vi "GUI.vi"() -> ()   [LabVIEW 2020]
uses:
  Sensor910/Sensor910.lvclass
  <vilib>/Utility/miscctls.llb/LVRectTypeDef.ctl
  Sensor910/Settings.ctl
  Sensor910/Mode.ctl
  Sensor910/Command.ctl
panel:
  in  "View Square":bool
  out "График температуры":sgl(graph)
  out "Connection":bool caption="Подключение"
  out "Tab Control":enum32{"Параметры", "Работа"}(tab)
  in  "h reg":u16=48 caption="Регистр h"
  in  "Modbus h":u8=240 caption="Адрес Modbus (Эталон H)"
  in  "dopusk":sgl=0.2 caption="Допуск погрешности, °С"
  in  "Temp Register 2":u8=2 caption="Регистр t (Эталон Т)"
  in  "Period":i64=100 caption="Частота опроса, мс"
  in  "Modbus t":u8=200 caption="Адрес Modbus (Эталон Т)"
  in  "Baud Rate":u32(ring)=9600 caption="Скорость обмена" items=["2400"=2400, "4800"=4800, "9600"=9600, "14400"=14400, "19200"=19200, "38400"=38400, "56000"=56000]
  in  "PIN":string="2210" caption="ПИН-код"
  in  "Modbus":u8=1 caption="Адрес Modbus"
  in  "Device":refnum<visa-resource-name> caption="Устройство"
  in  "Connect":bool
  in  "Pres Register":u16 caption="Регистр p"
  in  "Temp Register":u16=12 caption="Регистр t"
  out "Tab Control 3":enum32{"Температура", "Влажность", "Давление"}(tab)
  in  "temp tab":T1(tab)
  out "Current Offset":sgl caption="Текущее смещение температуры"
  in  "t_offset":i16 caption="Новое смещение температуры (0.1 °С)"
  in  "change offset t":bool
  out "Etalon temp":sgl caption="Температура (эталон, °С)"
  in  "humidity tab":T1(tab)
  out "Current Offset h":sgl caption="Текущее смещение влажности"
  in  "h_offset":i16 caption="Новое смещение влажности (0.01 %)"
  in  "change offset h":bool
  out "Etalon h":sgl caption="Влажность (эталон, %)"
  in  "press tab":T1(tab)
  out "Current Offset 3":sgl caption="Текущее смещение температуры"
  in  "t_offset 3":i16 caption="Новое смещение температуры (0.1 °С)"
  in  "change offset 3":bool
  out "Etalon temp 3":sgl caption="Температура (эталон, °С)"
  in  "Калибруемый параметр":enum16{"Температура", "Влажность", "Давление"}(ring)
  out "Pict Ring":u16(ring)
  out "Current Modbus":sgl caption="Текущий адрес Modbus"
  in  "Update Modbus Address":bool
  in  "New Modbus Address":u16=1 caption="Новый адрес Modbus"
  out "No Respose":bool
  in  "Disconnect":bool
  out "T 2":sgl caption="э t" format="%.3f"
  out "T":sgl caption="d t" format="%.3f"
  out "h 910":sgl caption="d h" format="%.3f"
  out "P":sgl caption="d p" format="%.3f"
  out "etalon h":sgl caption="э t" format="%.3f"
  # "Настройки подключения"
  # "Датчик"
  # "Эталон"
  # "Температура, °С"
  # "Влажность, %"
  # "Давление, Бар"
  # "Настройка Modbus"
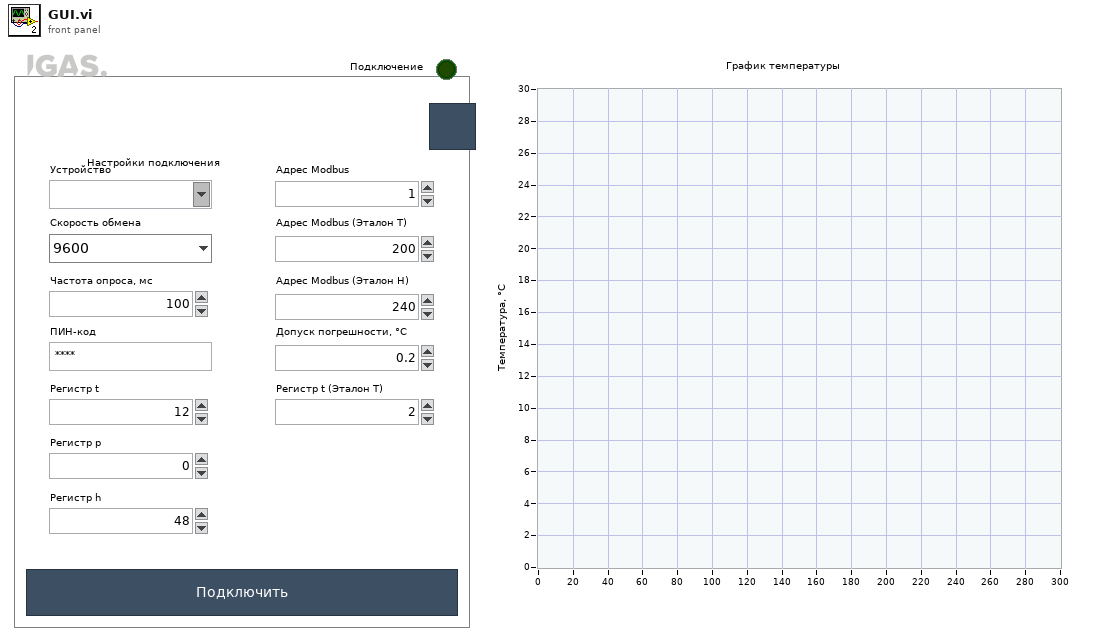
[diagram p1: front panel]
types:
  T1 = enum32{"Ручная калибровка", "Калибровка по эталону"}
  T2 = typedef "LVRectTypeDef.ctl" = cluster{"Left":i16, "Top":i16, "Right":i16, "Bottom":i16}
  T3 = typedef "Sensor910.lvclass/Mode.ctl" = enum16{"Inactiv", "Read Data", "Service Mode", "Enter offset", "Open session", "Close session", "Set Modbus Address", "Abort"}
  T4 = typedef "Sensor910.lvclass/Settings.ctl" = cluster{"Serial Parameters":cluster{"Mode":enum16{"RTU", "ASCII"}, "Slave Address":u8}, "VISA resource name":refnum<visa-resource-name>, "Period":i64, "Data Registers":u16[], "Baud Rate":u32}
  T5 = typedef "Sensor910.lvclass/Command.ctl" = cluster{"Address":u16, "Data":u16}
  T6 = typedef "Sensor910.lvclass/Data.ctl" = cluster{"Connect":bool, "No Response":bool, "Data":sgl[]}
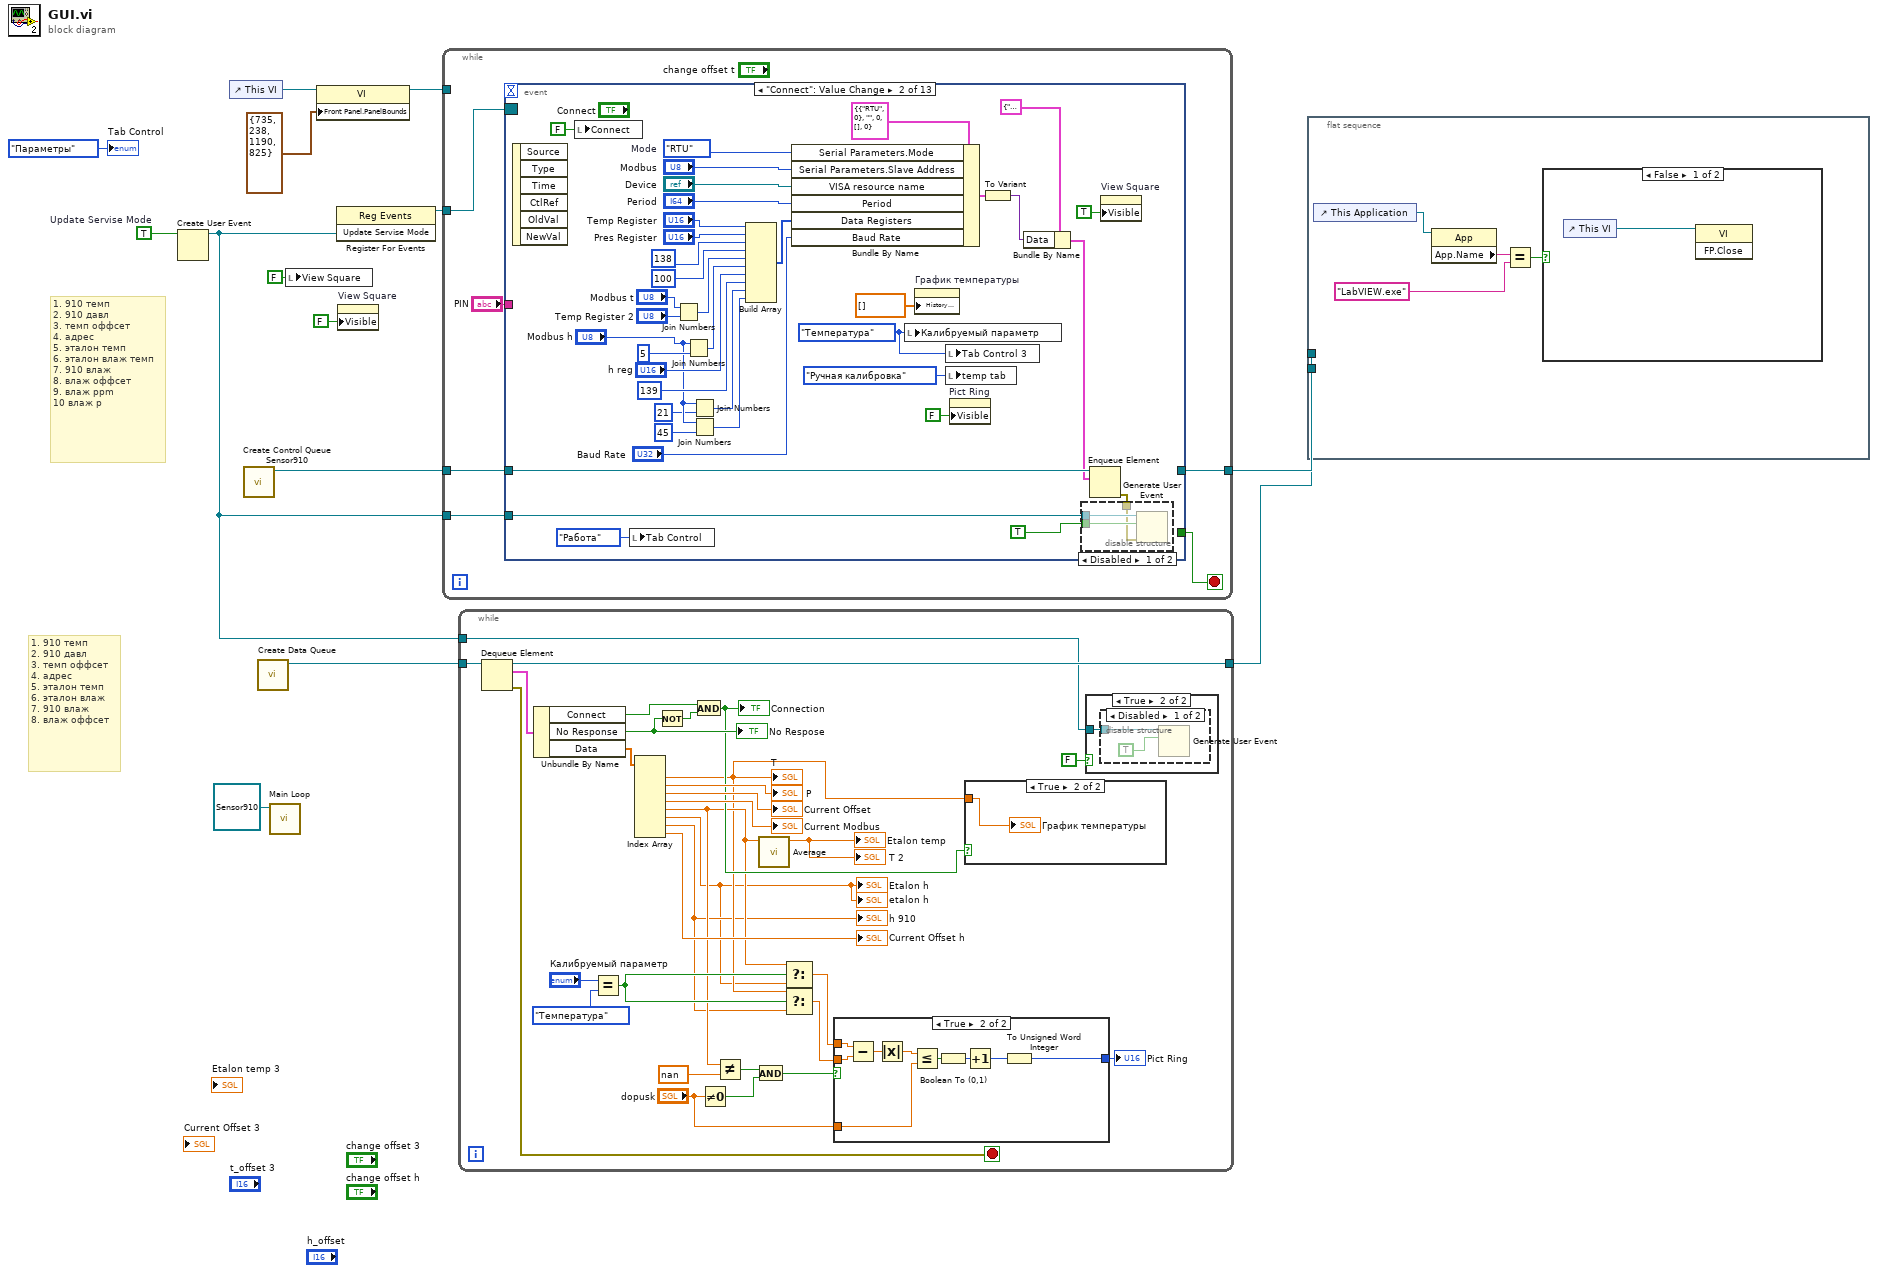
[diagram p0: block diagram]
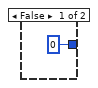
[diagram p4: hidden frame]
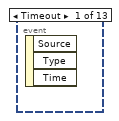
[diagram p7: hidden frame]
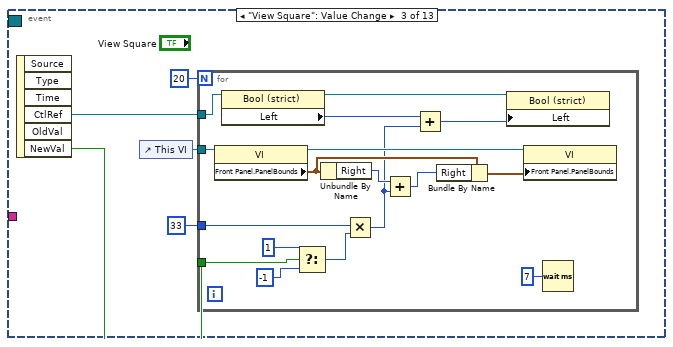
[diagram p9: hidden frame]
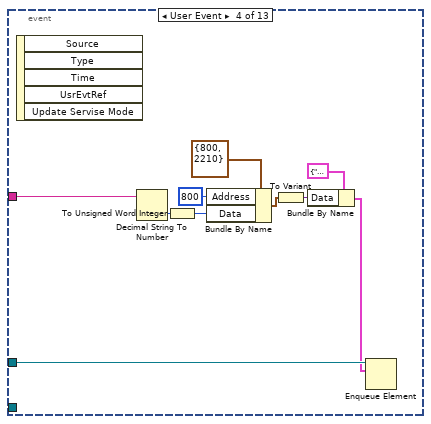
[diagram p10: hidden frame]
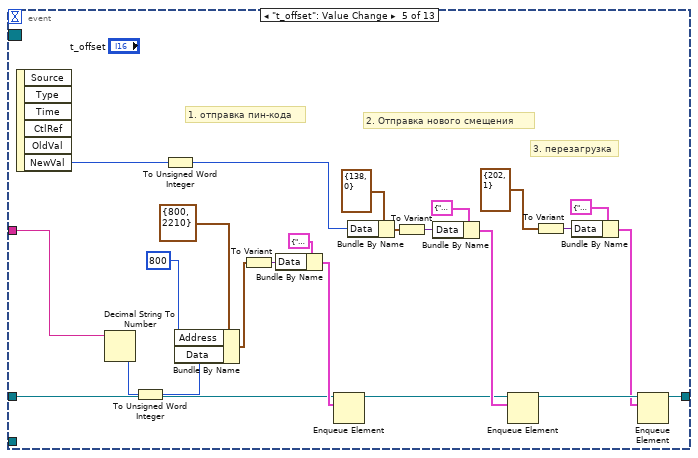
[diagram p11: hidden frame]
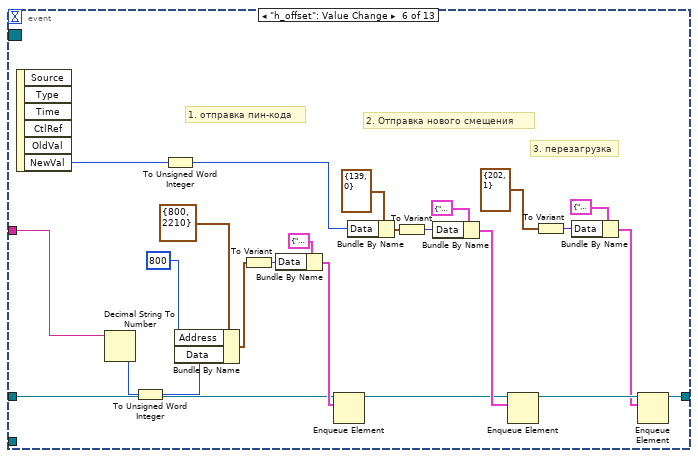
[diagram p12: hidden frame]
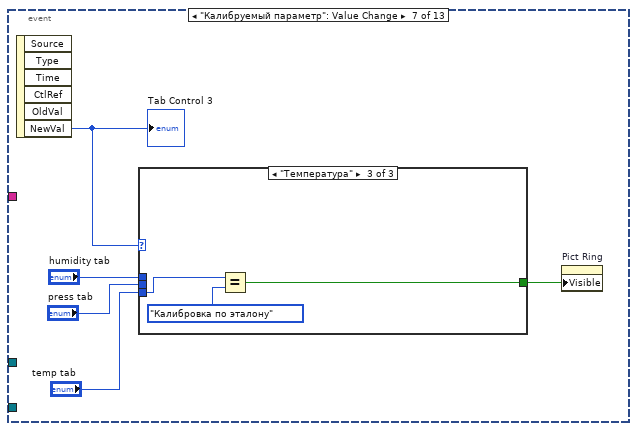
[diagram p13: hidden frame]
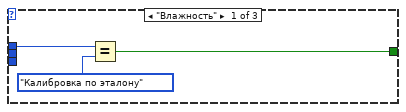
[diagram p14: hidden frame]
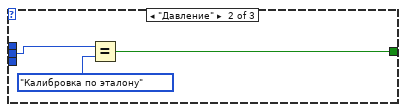
[diagram p15: hidden frame]
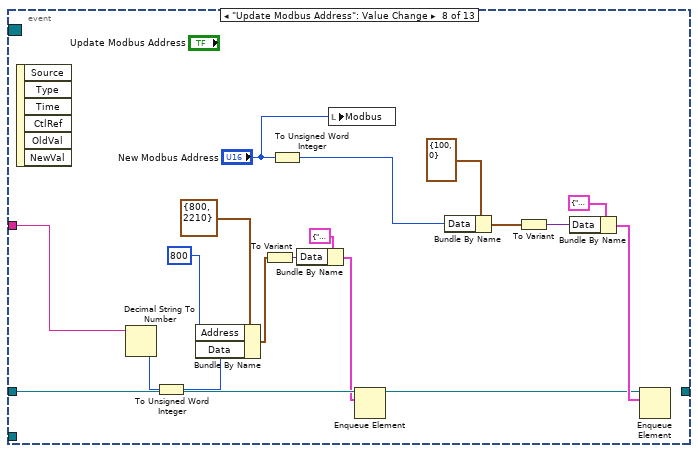
[diagram p16: hidden frame]
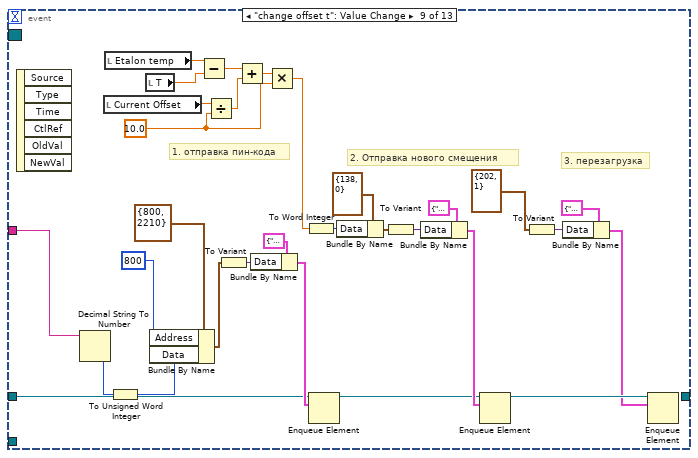
[diagram p17: hidden frame]
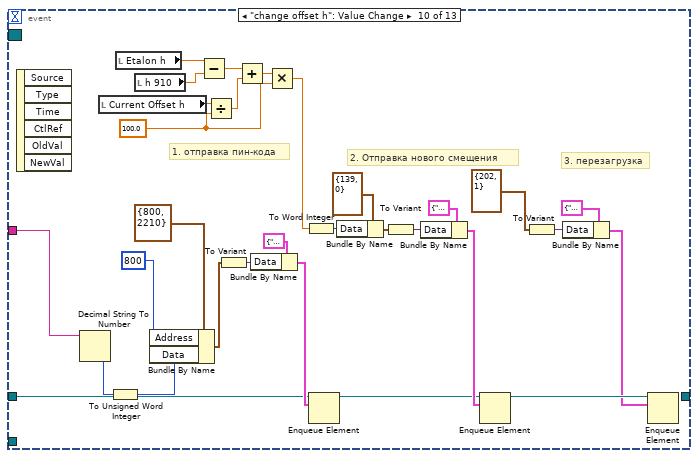
[diagram p18: hidden frame]
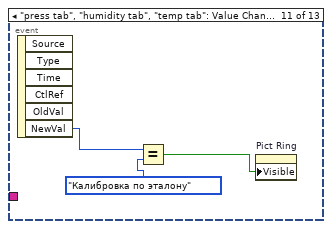
[diagram p19: hidden frame]
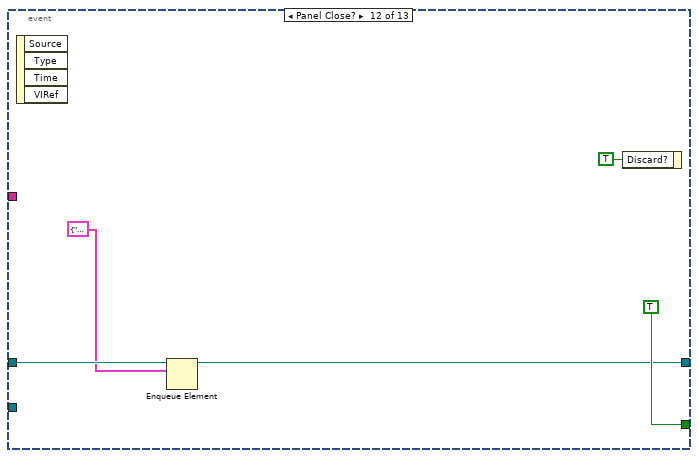
[diagram p20: hidden frame]
diagram:
  w8 = TRUE  # Update Servise Mode
  # "1. 910 темп\n2. 910 давл\n3. темп оффсет\n4. адрес\n5. эталон темп\n6. эталон влаж темп\n7. 910 влаж\n8. влаж оффсет\n9. влаж ppm\n10 влаж p"
  # "1. 910 темп\n2. 910 давл\n3. темп оффсет\n4. адрес\n5. эталон темп\n6. эталон влаж\n7. 910 влаж\n8. влаж оффсет"
  n1 = Create User Event(user event datatype=w8) -> (user event=w6:refnum<user-event>)  [unwired: 1 in, 1 out]
  n2 = control-ref of="This VI"() -> (w5:refnum<vi>)
  n3 = call "Create Control Queue Sensor910.vi"() -> ("queue out"=w14:refnum<queue>)  [unwired: 9 in, 2 out]
  n4 = call "Create Data Queue.vi"() -> ("queue out"=w13:refnum<queue>)  [unwired: 10 in, 1 out]
  n5 = call-dynamic "Main Loop.vi"("Sensor910 in"=refnum<class "Sensor910.lvclass"> refnum) -> ()  [unwired: 9 in, 2 out]
  n6 = local write "View Square"(FALSE ("Checkbox")) -> ()
  n7 = property class="VI"(reference=w5, "Front Panel.PanelBounds"=T2 {"Left"=735, "Top"=238, "Right"=1190, "Bottom"=825} ("Front Panel Window:Panel Bounds")) -> (reference out=w3:refnum<vi>)  [unwired: 1 in, 1 out]
  n8 = register-events(w6) -> (reference out=w7:refnum<event-registration>)  [unwired: 2 in, 1 out]
  n9 = property on="View Square" class="Bool (strict)"("Visible"=FALSE) -> ()  [unwired: 2 in, 2 out]
  n10 = while {
    tunnel: w14 -> [w20]
    tunnel: [w18] -> w11
    tunnel: w7 -> [w16]
    tunnel: w6 -> [w15]
    tunnel: w3 -> [_]
    stop <- w19 stop-if-true
    n11 = event shown="[1] \"Connect\": Value Change" {
      selector: w16 -> [_ _ _ _ _ _ _ _ _ _ _ _ _]
      dyn-events: _ -> [_ _ _ _ _ _ _ _ _ _ _ _ _]
      timeout: _ -> [_ _ _ _ _ _ _ _ _ _ _ _ _]
      tunnel: w20 -> [_ w37 _ w85 w96 w120 _ w160 w176 w206 _ w239 w245]
      tunnel: [_ _ _ _ _ _ _ _ _ _ _ TRUE _] -> w19
      tunnel: [_ _ _ _ w106 w130 _ _ _ _ _ w238 _] -> w18
      tunnel: "PIN" -> [_ _ _ w86 w94 w118 _ w159 w174 w204 _ _ _]
      tunnel: w15 -> [_ w44 _ _ _ _ _ _ _ _ _ _ _]
      event Timeout {
        n12 = event-data() -> ()  [unwired: 1 in, 3 out]
      }
      event "Connect": Value Change {
        w29 = enum16{"Температура", "Влажность", "Давление"}."Температура" ("Калибруемый параметр")
        w49 = enum16{"RTU", "ASCII"}."RTU"  # Mode
        n13 = event-data() -> ()  [unwired: 1 in, 6 out]
        n14 = local write "Connect"(FALSE ("Connect")) -> ()
        n15 = local write "Tab Control"(enum32{"Параметры", "Работа"}."Работа" ("Tab Control")) -> ()
        n16 = Join Numbers(hi="Modbus t", lo="Temp Register 2") -> ((hi.lo)=w38:u16)
        n17 = Join Numbers(hi="Modbus h", lo=u8 5) -> ((hi.lo)=w32:u16)
        n18 = Join Numbers(hi="Modbus h", lo=u8 21) -> ((hi.lo)=w22:u16)
        n19 = Join Numbers(hi="Modbus h", lo=u8 45) -> ((hi.lo)=w21:u16)
        n20 = Build Array("Temp Register", "Pres Register", u16 138 ("element"), u16 100 ("element"), w38, w32, "h reg", u16 139 ("element"), w22, w21) -> (w51:u16[])
        n21 = Bundle By Name(cluster=T4 {"Serial Parameters"={"Mode"=enum."RTU", "Slave Address"=0}, "VISA resource name"="", "Period"=0, "Data Registers"=[], "Baud Rate"=0} ("Cluster"), "Serial Parameters.Mode"=w49, "Serial Parameters.Slave Address"="Modbus", "VISA resource name"="Device", "Period"="Period", "Data Registers"=w51, "Baud Rate"="Baud Rate") -> (w41:T4)
        n22 = local write "Калибруемый параметр"(w29) -> ()
        n23 = property on="График температуры" class="WFChart (strict)"("History Data"=sgl[] []) -> ()  [unwired: 2 in, 2 out]
        n24 = local write "Tab Control 3"(w29) -> ()
        n25 = local write "temp tab"(T1."Ручная калибровка" ("temp tab")) -> ()
        n26 = property on="Pict Ring" class="Ring (strict)"("Visible"=FALSE) -> ()  [unwired: 2 in, 2 out]
        n27 = To Variant(anything=w41) -> (Variant=w56:variant)
        n28 = Bundle By Name(cluster=cluster{"Mode":T3, "Data":variant} {"Mode"=enum."Open session", "Data"=variant} ("notification"), "Data"=w56) -> (w35:cluster{"Mode":T3, "Data":variant})
        n29 = Enqueue Element(queue=w37, element=w35) -> (error out=w36:errorcluster)  [unwired: 2 in, 2 out]
        n30 = disable-structure shown="Disabled" {
          disable-tunnel: w44 -> [w61 _]
          disable-tunnel: TRUE ("event data") -> [w60 _]
          disable-tunnel: w36 -> [w59 _]
          frame Disabled {
            n31 = Generate User Event(user event=w61, event data cluster=w60, error in=w59) -> ()  [unwired: 1 in, 2 out]
          }
          frame Enabled {
          }
        }
        n32 = property on="View Square" class="Bool (strict)"("Visible"=TRUE) -> ()  [unwired: 2 in, 2 out]
      }
      event "View Square": Value Change {
        n33 = event-data() -> ("CtlRef"=w62:refnum<vi>, "NewVal"=w65:bool)  [unwired: 1 in, 4 out]
        n34 = control-ref of="This VI"() -> (w66:refnum<vi>)
        n35 = for {
          N: 20 -> [_]
          tunnel: w66 -> [w83]
          tunnel: w65 -> [w74]
          tunnel: i16 33 ("Right") -> [w73]
          tunnel: w62 -> [w71]
          n36 = property class="VI"(reference=w83) -> (reference out=w82:refnum<vi>, "Front Panel.PanelBounds"=w80:T2)  [unwired: 1 in, 1 out]
          n37 = property class="Bool (strict)"(reference=w71) -> (reference out=w70:refnum<vi>, "Left"=w69:i32)  [unwired: 1 in, 1 out]
          n38 = Select(t=i16 1 ("Right"), s=w74, f=i16 -1 ("Right")) -> (s? t:f=w77:i16)
          n39 = Unbundle By Name(w80) -> ("Right"=w81:i16)
          n40 = Multiply(x=w73, y=w77) -> (x*y=w68:i16)
          n41 = Add(x=w81, y=w68) -> (x+y=w79:i16)
          n42 = Add(x=w69, y=w68) -> (x+y=w67:i32)
          n43 = Bundle By Name(cluster=w80, "Right"=w79) -> (w78:T2)
          n44 = property class="Bool (strict)"(reference=w70, "Left"=w67) -> ()  [unwired: 1 in, 2 out]
          n45 = property class="VI"(reference=w82, "Front Panel.PanelBounds"=w78) -> ()  [unwired: 1 in, 2 out]
          n46 = Wait (ms)(milliseconds to wait=u32 7) -> ()  [unwired: 1 out]
        }
      }
      event User Event {
        n47 = event-data() -> ()  [unwired: 1 in, 5 out]
        n48 = Decimal String To Number(string=w86) -> (number=w88:i32)  [unwired: 2 in, 1 out]
        n49 = To Unsigned Word Integer(number=w88) -> (unsigned 16bit integer=w87:u16)
        n50 = Bundle By Name(cluster=T5 {"Address"=800, "Data"=2210} ("Command"), "Address"=u16 800, "Data"=w87) -> (w90:T5)
        n51 = To Variant(anything=w90) -> (Variant=w92:variant)
        n52 = Bundle By Name(cluster=cluster{"Mode":T3, "Data":variant} {"Mode"=enum."Service Mode", "Data"=variant} ("notification"), "Data"=w92) -> (w84:cluster{"Mode":T3, "Data":variant})
        n53 = Enqueue Element(queue=w85, element=w84) -> ()  [unwired: 2 in, 3 out]
      }
      event "t_offset": Value Change {
        # "3. перезагрузка"
        # "2. Отправка нового смещения"
        # "1. отправка пин-кода"
        n54 = event-data() -> ("NewVal"=w113:i16)  [unwired: 1 in, 5 out]
        n55 = Decimal String To Number(string=w94) -> (number=w99:i32)  [unwired: 2 in, 1 out]
        n56 = To Unsigned Word Integer(number=w99) -> (unsigned 16bit integer=w98:u16)
        n57 = To Unsigned Word Integer(number=w113) -> (unsigned 16bit integer=w105:u16)
        n58 = Bundle By Name(cluster=T5 {"Address"=800, "Data"=2210} ("Command"), "Address"=u16 800, "Data"=w98) -> (w101:T5)
        n59 = To Variant(anything=w101) -> (Variant=w103:variant)
        n60 = Bundle By Name(cluster=cluster{"Mode":T3, "Data":variant} {"Mode"=enum."Service Mode", "Data"=variant} ("notification"), "Data"=w103) -> (w97:cluster{"Mode":T3, "Data":variant})
        n61 = Enqueue Element(queue=w96, element=w97) -> (queue out=w95:refnum<queue>)  [unwired: 2 in, 2 out]
        n62 = Bundle By Name(cluster=T5 {"Address"=138, "Data"=0} ("Command"), "Data"=w105) -> (w114:T5)
        n63 = To Variant(anything=w114) -> (Variant=w117:variant)
        n64 = Bundle By Name(cluster=cluster{"Mode":T3, "Data":variant} {"Mode"=enum."Service Mode", "Data"=variant} ("notification"), "Data"=w117) -> (w109:cluster{"Mode":T3, "Data":variant})
        n65 = Enqueue Element(queue=w95, element=w109) -> (queue out=w108:refnum<queue>)  [unwired: 2 in, 2 out]
        n66 = To Variant(anything=T5 {"Address"=202, "Data"=1} ("Command")) -> (Variant=w111:variant)
        n67 = Bundle By Name(cluster=cluster{"Mode":T3, "Data":variant} {"Mode"=enum."Service Mode", "Data"=variant} ("notification"), "Data"=w111) -> (w107:cluster{"Mode":T3, "Data":variant})
        n68 = Enqueue Element(queue=w108, element=w107) -> (queue out=w106:refnum<queue>)  [unwired: 2 in, 2 out]
      }
      event "h_offset": Value Change {
        # "3. перезагрузка"
        # "2. Отправка нового смещения"
        # "1. отправка пин-кода"
        n69 = event-data() -> ("NewVal"=w137:i16)  [unwired: 1 in, 5 out]
        n70 = Decimal String To Number(string=w118) -> (number=w123:i32)  [unwired: 2 in, 1 out]
        n71 = To Unsigned Word Integer(number=w123) -> (unsigned 16bit integer=w122:u16)
        n72 = To Unsigned Word Integer(number=w137) -> (unsigned 16bit integer=w129:u16)
        n73 = Bundle By Name(cluster=T5 {"Address"=800, "Data"=2210} ("Command"), "Address"=u16 800, "Data"=w122) -> (w125:T5)
        n74 = To Variant(anything=w125) -> (Variant=w127:variant)
        n75 = Bundle By Name(cluster=cluster{"Mode":T3, "Data":variant} {"Mode"=enum."Service Mode", "Data"=variant} ("notification"), "Data"=w127) -> (w121:cluster{"Mode":T3, "Data":variant})
        n76 = Enqueue Element(queue=w120, element=w121) -> (queue out=w119:refnum<queue>)  [unwired: 2 in, 2 out]
        n77 = Bundle By Name(cluster=T5 {"Address"=139, "Data"=0} ("Command"), "Data"=w129) -> (w138:T5)
        n78 = To Variant(anything=w138) -> (Variant=w141:variant)
        n79 = Bundle By Name(cluster=cluster{"Mode":T3, "Data":variant} {"Mode"=enum."Service Mode", "Data"=variant} ("notification"), "Data"=w141) -> (w133:cluster{"Mode":T3, "Data":variant})
        n80 = Enqueue Element(queue=w119, element=w133) -> (queue out=w132:refnum<queue>)  [unwired: 2 in, 2 out]
        n81 = To Variant(anything=T5 {"Address"=202, "Data"=1} ("Command")) -> (Variant=w135:variant)
        n82 = Bundle By Name(cluster=cluster{"Mode":T3, "Data":variant} {"Mode"=enum."Service Mode", "Data"=variant} ("notification"), "Data"=w135) -> (w131:cluster{"Mode":T3, "Data":variant})
        n83 = Enqueue Element(queue=w132, element=w131) -> (queue out=w130:refnum<queue>)  [unwired: 2 in, 2 out]
      }
      event "Калибруемый параметр": Value Change {
        n84 = event-data() -> ("NewVal"=w146:enum16{"Температура", "Влажность", "Давление"})  [unwired: 1 in, 5 out]
        "Tab Control 3" <- w146
        n85 = case shown="\"Температура\"" w146 {
          tunnel: "humidity tab" -> [w149 _ _]
          tunnel: [w147 w151 w154] -> w144
          tunnel: "press tab" -> [_ w150 _]
          tunnel: "temp tab" -> [_ _ w153]
          frame "Влажность" {
            n86 = Equal?(x=w149, y=T1."Калибровка по эталону") -> (x = y?=w147:bool)
          }
          frame "Давление" {
            n87 = Equal?(x=w150, y=T1."Калибровка по эталону") -> (x = y?=w151:bool)
          }
          frame "Температура" {
            n88 = Equal?(x=w153, y=T1."Калибровка по эталону") -> (x = y?=w154:bool)
          }
        }
        n89 = property on="Pict Ring" class="Ring (strict)"("Visible"=w144) -> ()  [unwired: 2 in, 2 out]
      }
      event "Update Modbus Address": Value Change {
        n90 = event-data() -> ()  [unwired: 1 in, 6 out]
        n91 = Decimal String To Number(string=w159) -> (number=w162:i32)  [unwired: 2 in, 1 out]
        n92 = To Unsigned Word Integer(number=w162) -> (unsigned 16bit integer=w161:u16)
        n93 = Bundle By Name(cluster=T5 {"Address"=800, "Data"=2210} ("Command"), "Address"=u16 800, "Data"=w161) -> (w164:T5)
        n94 = To Variant(anything=w164) -> (Variant=w166:variant)
        n95 = To Unsigned Word Integer(number="New Modbus Address") -> (unsigned 16bit integer=w169:u16)
        n96 = Bundle By Name(cluster=cluster{"Mode":T3, "Data":variant} {"Mode"=enum."Service Mode", "Data"=variant} ("notification"), "Data"=w166) -> (w158:cluster{"Mode":T3, "Data":variant})
        n97 = local write "Modbus"("New Modbus Address") -> ()
        n98 = Enqueue Element(queue=w160, element=w158) -> (queue out=w156:refnum<queue>)  [unwired: 2 in, 2 out]
        n99 = Bundle By Name(cluster=T5 {"Address"=100, "Data"=0} ("Command"), "Data"=w169) -> (w170:T5)
        n100 = To Variant(anything=w170) -> (Variant=w173:variant)
        n101 = Bundle By Name(cluster=cluster{"Mode":T3, "Data":variant} {"Mode"=enum."Service Mode", "Data"=variant} ("notification"), "Data"=w173) -> (w167:cluster{"Mode":T3, "Data":variant})
        n102 = Enqueue Element(queue=w156, element=w167) -> ()  [unwired: 2 in, 3 out]
      }
      event "change offset t": Value Change {
        w187 = sgl 10.0 ("y")
        # "3. перезагрузка"
        # "2. Отправка нового смещения"
        # "1. отправка пин-кода"
        n103 = event-data() -> ()  [unwired: 1 in, 6 out]
        n104 = Decimal String To Number(string=w174) -> (number=w180:i32)  [unwired: 2 in, 1 out]
        n105 = local read "Current Offset"() -> (w189:sgl)
        n106 = local read "Etalon temp"() -> (w197:sgl)
        n107 = To Unsigned Word Integer(number=w180) -> (unsigned 16bit integer=w179:u16)
        n108 = local read "T"() -> (w196:sgl)
        n109 = Bundle By Name(cluster=T5 {"Address"=800, "Data"=2210} ("Command"), "Address"=u16 800, "Data"=w179) -> (w182:T5)
        n110 = Subtract(x=w197, y=w196) -> (x-y=w192:sgl)
        n111 = Divide(x=w189, y=w187) -> (x/y=w188:sgl)
        n112 = To Variant(anything=w182) -> (Variant=w184:variant)
        n113 = Add(x=w192, y=w188) -> (x+y=w191:sgl)
        n114 = Bundle By Name(cluster=cluster{"Mode":T3, "Data":variant} {"Mode"=enum."Service Mode", "Data"=variant} ("notification"), "Data"=w184) -> (w178:cluster{"Mode":T3, "Data":variant})
        n115 = Multiply(x=w191, y=w187) -> (x*y=w190:sgl)
        n116 = To Word Integer(number=w190) -> (16bit integer=w198:i16)
        n117 = Enqueue Element(queue=w176, element=w178) -> (queue out=w175:refnum<queue>)  [unwired: 2 in, 2 out]
        n118 = Bundle By Name(cluster=T5 {"Address"=138, "Data"=0} ("Command"), "Data"=w198) -> (w199:T5)
        n119 = To Variant(anything=w199) -> (Variant=w203:variant)
        n120 = Bundle By Name(cluster=cluster{"Mode":T3, "Data":variant} {"Mode"=enum."Service Mode", "Data"=variant} ("notification"), "Data"=w203) -> (w200:cluster{"Mode":T3, "Data":variant})
        n121 = Enqueue Element(queue=w175, element=w200) -> (queue out=w186:refnum<queue>)  [unwired: 2 in, 2 out]
        n122 = To Variant(anything=T5 {"Address"=202, "Data"=1} ("Command")) -> (Variant=w195:variant)
        n123 = Bundle By Name(cluster=cluster{"Mode":T3, "Data":variant} {"Mode"=enum."Service Mode", "Data"=variant} ("notification"), "Data"=w195) -> (w185:cluster{"Mode":T3, "Data":variant})
        n124 = Enqueue Element(queue=w186, element=w185) -> ()  [unwired: 2 in, 3 out]
      }
      event "change offset h": Value Change {
        w217 = sgl 100.0 ("y")
        # "3. перезагрузка"
        # "2. Отправка нового смещения"
        # "1. отправка пин-кода"
        n125 = event-data() -> ()  [unwired: 1 in, 6 out]
        n126 = Decimal String To Number(string=w204) -> (number=w210:i32)  [unwired: 2 in, 1 out]
        n127 = local read "Current Offset h"() -> (w219:sgl)
        n128 = To Unsigned Word Integer(number=w210) -> (unsigned 16bit integer=w209:u16)
        n129 = local read "Etalon h"() -> (w227:sgl)
        n130 = local read "h 910"() -> (w226:sgl)
        n131 = Bundle By Name(cluster=T5 {"Address"=800, "Data"=2210} ("Command"), "Address"=u16 800, "Data"=w209) -> (w212:T5)
        n132 = Subtract(x=w227, y=w226) -> (x-y=w222:sgl)
        n133 = Divide(x=w219, y=w217) -> (x/y=w218:sgl)
        n134 = To Variant(anything=w212) -> (Variant=w214:variant)
        n135 = Add(x=w222, y=w218) -> (x+y=w221:sgl)
        n136 = Bundle By Name(cluster=cluster{"Mode":T3, "Data":variant} {"Mode"=enum."Service Mode", "Data"=variant} ("notification"), "Data"=w214) -> (w208:cluster{"Mode":T3, "Data":variant})
        n137 = Multiply(x=w221, y=w217) -> (x*y=w220:sgl)
        n138 = To Word Integer(number=w220) -> (16bit integer=w228:i16)
        n139 = Enqueue Element(queue=w206, element=w208) -> (queue out=w205:refnum<queue>)  [unwired: 2 in, 2 out]
        n140 = Bundle By Name(cluster=T5 {"Address"=139, "Data"=0} ("Command"), "Data"=w228) -> (w229:T5)
        n141 = To Variant(anything=w229) -> (Variant=w233:variant)
        n142 = Bundle By Name(cluster=cluster{"Mode":T3, "Data":variant} {"Mode"=enum."Service Mode", "Data"=variant} ("notification"), "Data"=w233) -> (w230:cluster{"Mode":T3, "Data":variant})
        n143 = Enqueue Element(queue=w205, element=w230) -> (queue out=w216:refnum<queue>)  [unwired: 2 in, 2 out]
        n144 = To Variant(anything=T5 {"Address"=202, "Data"=1} ("Command")) -> (Variant=w225:variant)
        n145 = Bundle By Name(cluster=cluster{"Mode":T3, "Data":variant} {"Mode"=enum."Service Mode", "Data"=variant} ("notification"), "Data"=w225) -> (w215:cluster{"Mode":T3, "Data":variant})
        n146 = Enqueue Element(queue=w216, element=w215) -> ()  [unwired: 2 in, 3 out]
      }
      event "press tab", "humidity tab", "temp tab": Value Change {
        n147 = event-data() -> ("NewVal"=w236:T1)  [unwired: 1 in, 5 out]
        n148 = Equal?(x=w236, y=T1."Калибровка по эталону") -> (x = y?=w235:bool)
        n149 = property on="Pict Ring" class="Ring (strict)"("Visible"=w235) -> ()  [unwired: 2 in, 2 out]
      }
      event Panel Close? {
        n150 = event-data() -> ()  [unwired: 1 in, 4 out]
        n151 = Enqueue Element(queue=w239, element=cluster{"Mode":T3, "Data":variant} {"Mode"=enum."Abort", "Data"=variant} ("notification")) -> (queue out=w238:refnum<queue>)  [unwired: 2 in, 2 out]
        n152 = event-data("Discard?"=TRUE) -> ()  [unwired: 1 in, 1 out]
      }
      event "Disconnect": Value Change {
        n153 = event-data() -> ()  [unwired: 1 in, 6 out]
        n154 = local read "View Square"() -> (w243:bool)
        n155 = case shown="True" w243 {
          frame False {
          }
          frame True {
            n156 = control-ref of="View Square"() -> (w248:refnum<vi>)
            n157 = control-ref of="This VI"() -> (w250:refnum<vi>)
            n158 = for {
              N: 20 -> [_]
              tunnel: w250 -> [w263]
              tunnel: w248 -> [w252]
              w251 = i16 -33 ("Right")
              n159 = property class="VI"(reference=w263) -> (reference out=w262:refnum<vi>, "Front Panel.PanelBounds"=w260:T2)  [unwired: 1 in, 1 out]
              n160 = property class="Bool (strict)"(reference=w252) -> (reference out=w255:refnum<vi>, "Left"=w254:i32)  [unwired: 1 in, 1 out]
              n161 = Unbundle By Name(w260) -> ("Right"=w261:i16)
              n162 = Add(x=w261, y=w251) -> (x+y=w259:i16)
              n163 = Add(x=w254, y=w251) -> (x+y=w253:i32)
              n164 = local write "View Square"(FALSE ("Checkbox")) -> ()
              n165 = Bundle By Name(cluster=w260, "Right"=w259) -> (w258:T2)
              n166 = property class="Bool (strict)"(reference=w255, "Left"=w253) -> ()  [unwired: 1 in, 2 out]
              n167 = property class="VI"(reference=w262, "Front Panel.PanelBounds"=w258) -> ()  [unwired: 1 in, 2 out]
              n168 = Wait (ms)(milliseconds to wait=u32 7) -> ()  [unwired: 1 out]
            }
          }
        }
        n169 = local write "Tab Control"(enum32{"Параметры", "Работа"}."Параметры" ("Tab Control")) -> ()
        n170 = Enqueue Element(queue=w245, element=cluster{"Mode":T3, "Data":variant} {"Mode"=enum."Close session", "Data"=variant} ("notification")) -> ()  [unwired: 2 in, 3 out]
        n171 = local write "Disconnect"(FALSE ("Disconnect")) -> ()
        n172 = property on="View Square" class="Bool (strict)"("Visible"=FALSE) -> ()  [unwired: 2 in, 2 out]
      }
    }
  }
  n173 = while {
    tunnel: w13 -> [w294]
    tunnel: [w289] -> w10
    tunnel: w6 -> [w287]
    stop <- w293 stop-if-true
    n174 = Dequeue Element(queue=w294) -> (queue out=w289:refnum<queue>, element=w292:T6, error out=w293:errorcluster)  [unwired: 2 in, 1 out]
    n175 = Unbundle By Name(w292) -> ("Connect"=w285:bool, "No Response"=w284:bool, "Data"=w291:sgl[])
    "No Respose" <- w284
    n176 = Equal?(x="Калибруемый параметр", y=enum16{"Температура", "Влажность", "Давление"}."Температура") -> (x = y?=w270:bool)
    n177 = Index Array(array=w291) -> (element #1=w268:sgl, element #2=→"P":sgl, element #3=→"Current Offset":sgl, element #4=→"Current Modbus":sgl, element #5=w269:sgl, element #6=w265:sgl, element #7=w266:sgl, element #8=→"Current Offset h":sgl)  [unwired: 8 in]
    "T" <- w268
    "Etalon h" <- w265
    "etalon h" <- w265
    "h 910" <- w266
    n178 = Not(x=w284) -> (.not. x?=w276:bool)
    n179 = And(x=w285, y=w276) -> (x .and. y?=w275:bool)
    "Connection" <- w275
    n180 = Not Equal To 0?(x="dopusk") -> (x != 0?=w280:bool)
    n181 = Not Equal?(x=w269, y=sgl nan) -> (x != y?=w281:bool)
    n182 = And(x=w281, y=w280) -> (x .and. y?=w279:bool)
    n183 = call "Average.vi"("p_atm"=w269) -> ("Average value"=→"Etalon temp" →"T 2":sgl)  [unwired: 10 in]
    n184 = Select(t=w269, s=w270, f=w265) -> (s? t:f=w267:sgl)
    n185 = Select(t=w268, s=w270, f=w266) -> (s? t:f=w264:sgl)
    n186 = case shown="True" w279 {
      tunnel: w264 -> [_ w305]
      tunnel: w267 -> [_ w304]
      tunnel: "dopusk" -> [_ w301]
      tunnel: [u16 0 w297] -> w278
      frame False {
      }
      frame True {
        n187 = Subtract(x=w304, y=w305) -> (x-y=w303:sgl)
        n188 = Absolute Value(x=w303) -> (abs(x)=w302:sgl)
        n189 = Less Or Equal?(x=w302, y=w301) -> (x <= y?=w300:bool)
        n190 = Boolean To (0,1)(Boolean=w300) -> (0, 1=w299:i16)
        n191 = Increment(x=w299) -> (x+1=w298:i16)
        n192 = To Unsigned Word Integer(number=w298) -> (unsigned 16bit integer=w297:u16)
      }
    }
    "Pict Ring" <- w278
    n193 = case shown="True" w275 {
      tunnel: w268 -> [_ w295]
      frame False {
      }
      frame True {
        "График температуры" <- w295
      }
    }
    n194 = case shown="True" FALSE {
      tunnel: w287 -> [_ w306]
      frame False {
      }
      frame True {
        n195 = disable-structure shown="Disabled" {
          disable-tunnel: w306 -> [w308 _]
          frame Disabled {
            n196 = Generate User Event(user event=w308, event data cluster=TRUE ("event data")) -> ()  [unwired: 2 in, 2 out]
          }
          frame Enabled {
          }
        }
      }
    }
  }
  n197 = flat-sequence {
    tunnel: w11 -> [_]
    tunnel: w10 -> [_]
    frame #0 {
      n198 = control-ref of="This Application"() -> (w312:refnum<vi>)
      n199 = property class="App"(reference=w312) -> ("App.Name"=w311:string)  [unwired: 1 in, 2 out]
      n200 = Equal?(x=w311, y="LabVIEW.exe") -> (x = y?=w309:bool)
      n201 = case shown="False" w309 {
        frame False {
          n202 = control-ref of="This VI"() -> (w313:refnum<vi>)
          n203 = invoke class="VI" method="FP.Close"(reference=w313) -> ()  [unwired: 2 in, 3 out]
        }
        frame True {
        }
      }
    }
  }
  "Tab Control" <- enum32{"Параметры", "Работа"}."Параметры" ("Tab Control")
